vi "Table-UpdateTBL.vi"(5 "Data for Front Panel Table":string[][](table), 7 "Column Headers":string[](array[string]), 8 "error in (no error)":errorcluster, 11 "ERP-SpecificationManager in":refnum<class "ERP-SpecificationManager.lvclass">) -> (0 "error out":errorcluster, 3 "ERP-SpecificationManager out":refnum<class "ERP-SpecificationManager.lvclass">)   [LabVIEW 2013, in "ERP-SpecificationManager.lvclass"]
uses:
  ERP-SpecificationManager.lvclass
  ERP-SpecificationManager.lvclass/ERP-SpecificationManager.ctl
  <vilib>/Utility/miscctls.llb/LVRowAndColumnUnsignedTypeDef.ctl
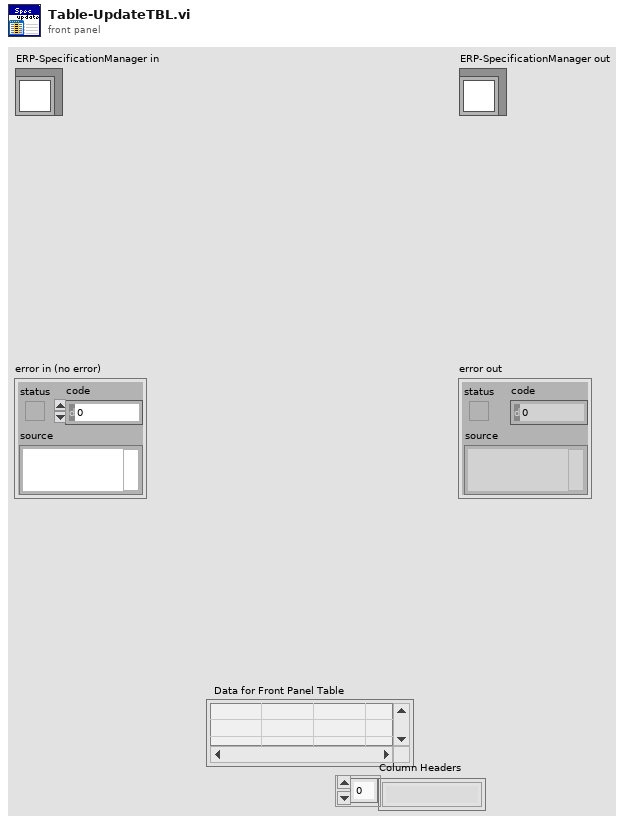
[diagram p1: front panel]
types:
  T1 = typedef "LVRowAndColumnUnsignedTypeDef.ctl" = cluster{"Row":u32, "Column":u32}
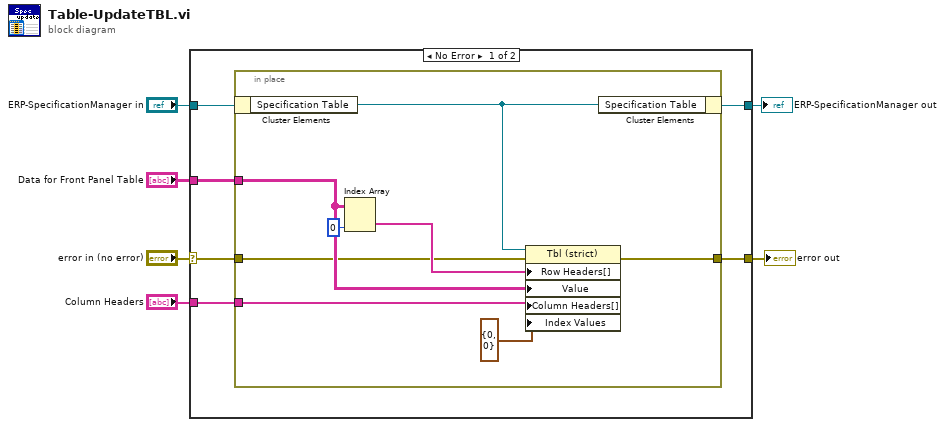
[diagram p0: block diagram]
diagram:
  n1 = case shown="No Error" "error in (no error)" {
    selector: "error in (no error)" -> [w8 w22]
    tunnel: [w7 w22] -> w5
    tunnel: [w9 w21] -> w3
    tunnel: "ERP-SpecificationManager in" -> [w10 w21]
    tunnel: "Column Headers" -> [w12 _]
    tunnel: "Data for Front Panel Table" -> [w11 _]
    frame No Error {
      n2 = in-place {
        in-place-border: w12 -> [w16]
        in-place-border: w11 -> [w15]
        in-place-border: w8 -> [w14]
        in-place-border: [w13] -> w7
        n3 = in-place-cluster #1(w10) -> ("Specification Table"=w17:refnum<vi>)
        n4 = Index Array(array=w15, index (col)=0 ("disabled index (col)")) -> (element=w19:string[])  [unwired: 1 in]
        n5 = property class="Tbl (strict)"(reference=w17, error in=w14, "Row Headers[]"=w19, "Value"=w15, "Column Headers[]"=w16, "Index Values"=T1 {"Row"=0, "Column"=0}) -> (error out=w13:errorcluster)  [unwired: 1 out]
        n6 = in-place-cluster #1("Specification Table"=w17) -> (w9:refnum<class "ERP-SpecificationManager.lvclass">)
      }
    }
    frame Error {
    }
  }
  "error out" <- w5
  "ERP-SpecificationManager out" <- w3
